vi "Lvi Set Shunt Resistor.vi"(8 "error in (no error)":errorcluster, 9 "ShuntEnabled":bool, 10 "Channel":u32, 11 "TaskRef":i32) -> (0 "error out":errorcluster, 2 "function return":u32(ring), 3 "TaskRef out":i32)   [LabVIEW 2022 SP3, in "DtLvLink.lvlib"]
doc: "Calls directly into the entry points of the DLL of the Data Acq SDK to enable or disable the shunt resistor for an analog input task. The shunt resistor is used when performing shunt calibration on a device that supports strain gage inputs or to verify the operation of your bridge. Refer to the documentation for your device for information on shunt calibration."
uses:
  DtLvLink.lvlib
  <userlib>/LV-Link3/DtLvLink_64.dll
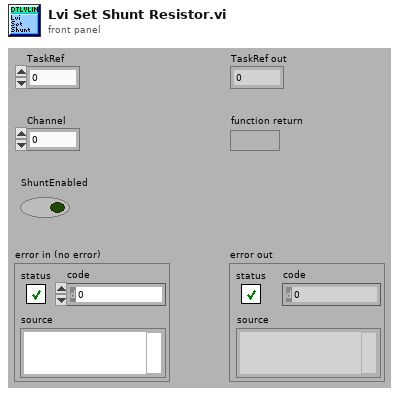
[diagram p1: front panel]
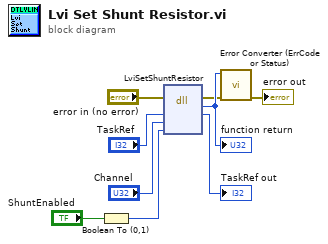
[diagram p0: block diagram]
diagram:
  n1 = Boolean To (0,1)(Boolean="ShuntEnabled") -> (0, 1=w4:i16)
  n2 = dll-call lib="C:/Program Files/National Instruments/LabVIEW 2022/user.lib/LV-Link3/DtLvLink_64.*" fn="LviSetShuntResistor"(error in="error in (no error)", "TaskRef"="TaskRef", "Channel"="Channel", "ShuntEnabled"=w4) -> (error out=w2:errorcluster, w9:u32, "TaskRef"=→"TaskRef out":i32)  [unwired: 4 in, 1 out]
  "function return" <- w9
  n3 = call "Error Converter (ErrCode or Status).vi"("error in (no error)"=w2, "error code"=w9) -> ("error out"=→"error out":errorcluster)  [unwired: 9 in]
